vi "Error Log Ref (class variable).vi"() -> ()   [LabVIEW 2016, in "Error Manager.lvlib" / "Error Log.lvclass"]
uses:
  Error Log.lvclass
panel:
  in  "Error Log Ref":refnum<file>
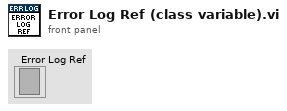
[diagram p1: front panel]
diagram:
